vi "格式时间字符串.vi"(11 "字符串":string) -> (3 "连接的字符串":string)   [LabVIEW 2016, in "数据传输系统-02.lvlib"]
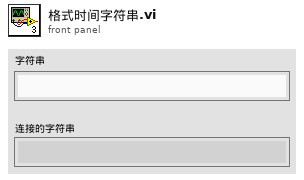
[diagram p1: front panel]
types:
  T1 = typedef "LVDateTimeRec.ctl" = cluster{"秒数的小数部分":dbl, "秒":i32, "分":i32, "时":i32, "日":i32, "月":i32, "年":i32, "天数（周）":i32, "天数（年）":i32, "DST":i32}
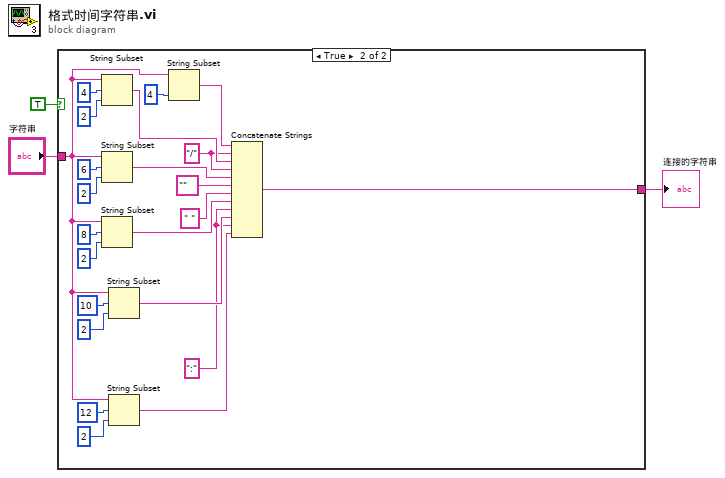
[diagram p0: block diagram]
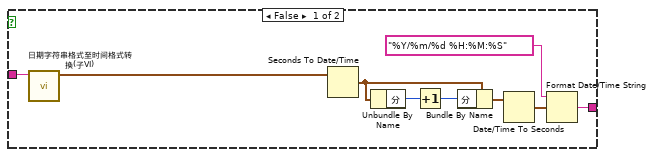
[diagram p2: hidden frame]
diagram:
  n1 = case shown="True" TRUE {
    tunnel: [w4 w16] -> w1
    tunnel: "字符串" -> [w5 w13]
    frame False {
      n2 = call "日期字符串格式至时间格式转换(子VI).vi"("data[0]"=w5) -> ("time stamp"=w6:timestamp)  [unwired: 10 in]
      n3 = Seconds To Date/Time(time stamp (now)=w6) -> (date time rec=w8:T1)  [unwired: 1 in]
      n4 = Unbundle By Name(w8) -> ("分"=w7:i32)
      n5 = Increment(x=w7) -> (x+1=w9:i32)
      n6 = Bundle By Name(cluster=w8, "分"=w9) -> (w11:T1)
      n7 = Date/Time To Seconds(2:w11) -> (0:w10:timestamp)  [unwired: 1 in]
      n8 = Format Date/Time String(time format string (%c)="%Y/%m/%d %H:%M:%S" ("时间格式字符串(%c)"), seconds (now)=w10) -> (date/time string=w4:string)  [unwired: 1 in]
    }
    frame True {
      w20 = ":" ("子字符串;substring")
      w25 = "/" ("子字符串;substring")
      n9 = String Subset(string=w13, offset (0)=4 ("偏移量(0)"), length (rest)=2 ("长度（剩余）")) -> (substring=w27:string)
      n10 = String Subset(string=w13, offset (0)=6 ("偏移量(0)"), length (rest)=2 ("长度（剩余）")) -> (substring=w26:string)
      n11 = String Subset(string=w13, offset (0)=8 ("偏移量(0)"), length (rest)=2 ("长度（剩余）")) -> (substring=w24:string)
      n12 = String Subset(string=w13, offset (0)=10 ("偏移量(0)"), length (rest)=2 ("长度（剩余）")) -> (substring=w21:string)
      n13 = String Subset(string=w13, offset (0)=12 ("偏移量(0)"), length (rest)=2 ("长度（剩余）")) -> (substring=w17:string)
      n14 = String Subset(string=w13, length (rest)=4 ("长度（剩余）")) -> (substring=w28:string)  [unwired: 1 in]
      n15 = Concatenate Strings(w28, w25, w27, w25, w26, "", " " ("子字符串;substring"), w24, w20, w21, w20, w17) -> (w16:string)
    }
  }
  "连接的字符串" <- w1
